vi "Plate Tank 5.vi"() -> ()   [LabVIEW 2019]
uses:
  <vilib>/NI/Current Value Table/Type Defs/Single Tag.ctl
  <vilib>/NI/Current Value Table/Type Defs/Data Types.ctl
  <vilib>/NI/STM/TCP/Read Meta Data (TCP Ref).vi
  <vilib>/NI/STM/TCP/Get Connection Reference (TCP).vi
  <vilib>/NI/AMC/Read Termination Message.vi
  <vilib>/NI/AMC/Create Single Message.vi
  <vilib>/NI/AMC/Update Message Routing Info.vi
  <vilib>/NI/STM/TCP/Read Meta Data (TCP Clst).vi
  <vilib>/NI/AMC/Send Message.vi
  <vilib>/NI/AMC/Globals.vi
  <userlib>/_OpenG.lib/comparison/comparison.llb/I32 Changed__ogtk.vi
  <vilib>/NI/STM/TCP/Write Message (TCP).vi
  <vilib>/NI/AMC/AMC.lvlib
  <vilib>/NI/STM/NI STM.lvlib
  <vilib>/NI/Current Value Table/Current Value Table.lvlib
panel:
  out "Loaded Recipe":string
  in  "Override Motion":bool
  in  "Reverse Current Multiplier":dbl=3.0 min=0.1 max=100.0 step=0.01 format="%.2g"
  in  "Load A Recipe":bool
  in  "Save This Recipe":bool
  out "Right Time":dbl format="%.1f"
  out "Left Time":dbl format="%.1f"
  out "Total Amp*min R":dbl format="%.1f"
  out "Total Amp*min L":dbl format="%.1f"
  in  "Rectifer Settings":i32(listbox)
  in  "MO":string
  in  "BasT1_P Last Hr":bool
  in  "BasT1_Level Last Hr":bool
  out "Boolean 5":bool
  out "SumpBottom":bool
  out "Process 1 Supply":bool
  out "Sump Return":bool
  out "Boolean 2":bool
  out "SG":dbl format="%.3g"
  out "Return to sump 4":bool
  in  "Rectifer Data":enum32{"Standard", "Eng"}(tab)
  out "Current Step":i32
  out "Left Anode Actual Current":dbl(knob) scale=0.0..150.0
  out "Right Anode Actual Current":dbl(knob) scale=0.0..150.0
  out "Left Anode Amp-min":dbl(slide) scale=0.0..800.0
  out "Right Anode Amp-min":dbl(slide) scale=0.0..233.60000610351562
  out "Output Voltage":cluster{dbl, dbl}(graph)
  in  "Tab Control 2":enum32{"Standard", "ENG"}(tab)
  in  "Level Last Hr":bool
  out "Supply Flow":dbl(knob) scale=0.0..65.0
  out "Plating Cell Liquid Level":dbl(slide) scale=0.0..75.0
  out "Cell Temperature":dbl(slide) scale=0.0..60.0
  in  "Cell T Last Hr":bool
  out "Suck Pump":bool
  out "Suck Pump Flow":dbl format="%#_4g"
  out "SuckPipe":bool
  out "SuckPipe 3":bool
  out "Drain Tee Top":bool
  out "Return to sump 2":bool
  out "Return to sump 3":bool
  in  "Supply Tot FlwLast Hr":bool
  in  "Suck FlwLast Hr":bool
  out "Flow Controller":dbl(knob) scale=0.0..100.0
  in  "Tab Control":enum32{"Main Pump", "Suck Pump"}(tab)
  out "Amps":dbl format="%#.2g"
  out "Volts":dbl format="%#.1f"
  out "VFD T":dbl format="%#.2g"
  out "RPM":dbl format="%#.0f"
  out "Fault Code":dbl format="%#.2g"
  out "Freq":dbl format="%#.2g"
  out "SP1 Amps":dbl caption="Amps" format="%#.2g"
  out "SP1 Volts":dbl caption="Volts" format="%#.1g"
  out "SP1 RPM":dbl caption="RPM" format="%#.2g"
  out "SP1 VFD T":dbl caption="VFD T" format="%#.2g"
  out "SP1 Fault Code":dbl caption="Fault Code" format="%#.2g"
  out "SP1 Freq":dbl caption="Freq" format="%#.2g"
  out "Flow 1":dbl format="%#_4g"
  out "Flow 2":dbl format="%#_4g"
  out "Flow 3":dbl format="%#_4g"
  out "Flow 4":dbl format="%#_4g"
  in  "FlowControl Last Hr":bool
  in  "Flow 1 Last Hr":bool
  in  "Flow 2 Last Hr":bool
  in  "Flow 3 Last Hr":bool
  in  "Flow 4 Last Hr":bool
  out "Return to sump":bool
  out "E Stop":bool
  out "Run Enabled?":bool
  in  "Full Drain Plating Cell":bool
  out "Rack Motion":bool
  out "Right Eductor Motion":bool
  out "Left Eductor Motion":bool
  out "Right Output On":bool
  in  "Enable Rack Motion":bool
  in  "Rack RPM":dbl(knob) scale=0.0..15.0
  out "Left Output On":bool
  in  "Start Cycle":bool
  in  "Cancel Cycle":bool
  out "SuckPipe 2":bool
  out "Main Pump":bool
  in  "Enable Eductor Motion":bool
  in  "Eductor RPM":dbl(knob) scale=0.0..15.0
  in  "Supply Pressure (kPa)":dbl(knob)=50.0 min=50.0 max=200.0 step=5.0 scale=50.0..200.0
  in  "Total Inflow (L/min)":dbl(knob)=40.0 min=25.0 max=50.0 step=0.5 scale=25.0..50.0
  in  "Suck Pump fraction of inflow":dbl(knob)=5.0 min=5.0 max=90.0 step=1.0 scale=0.0..90.0
  out "Sump Level":dbl(slide) scale=0.0..1000.0
  out "Supply Pressure":dbl(knob) scale=0.0..200.0
  in  "Enable Suck Pump":bool
  in  "Enable Plating Cell":bool
  in  "Machine":bool
  in  "Basement 4":bool
  in  "Dryer":bool
  in  "Rinse 4":bool
  in  "Rinse 3":bool
  in  "Rinse 2":bool
  in  "Basement 3":bool
  in  "Basement 2":bool
  in  "Basement 1":bool
  in  "Plater 6":bool
  in  "Plater 5":bool
  in  "Plater 4":bool
  in  "Plater 3":bool
  in  "Plater 2":bool
  in  "Plater 1":bool
  in  "Predip":bool
  in  "Rinse 1":bool
  in  "Cleaner":bool
  in  "Etch":bool
  out "status":string
  out "Boolean 4":bool
  # "Module Selection"
  # "Rectifier Settings"
  # "Fluid Flow Control"
  # "Rectifier Control"
  # "Rectifier Output"
  # "Note: RPM settings shared with tank 6"
  # "Motion starts when rectifiers cycle"
  # "kPa"
  # "@"
  # "Output"
  # "cm"
  # "°C"
  # "L/min"
  # "cm"
  # "L/min"
  # "L/min"
  # "L/min"
  # "L/min"
  # "L/min"
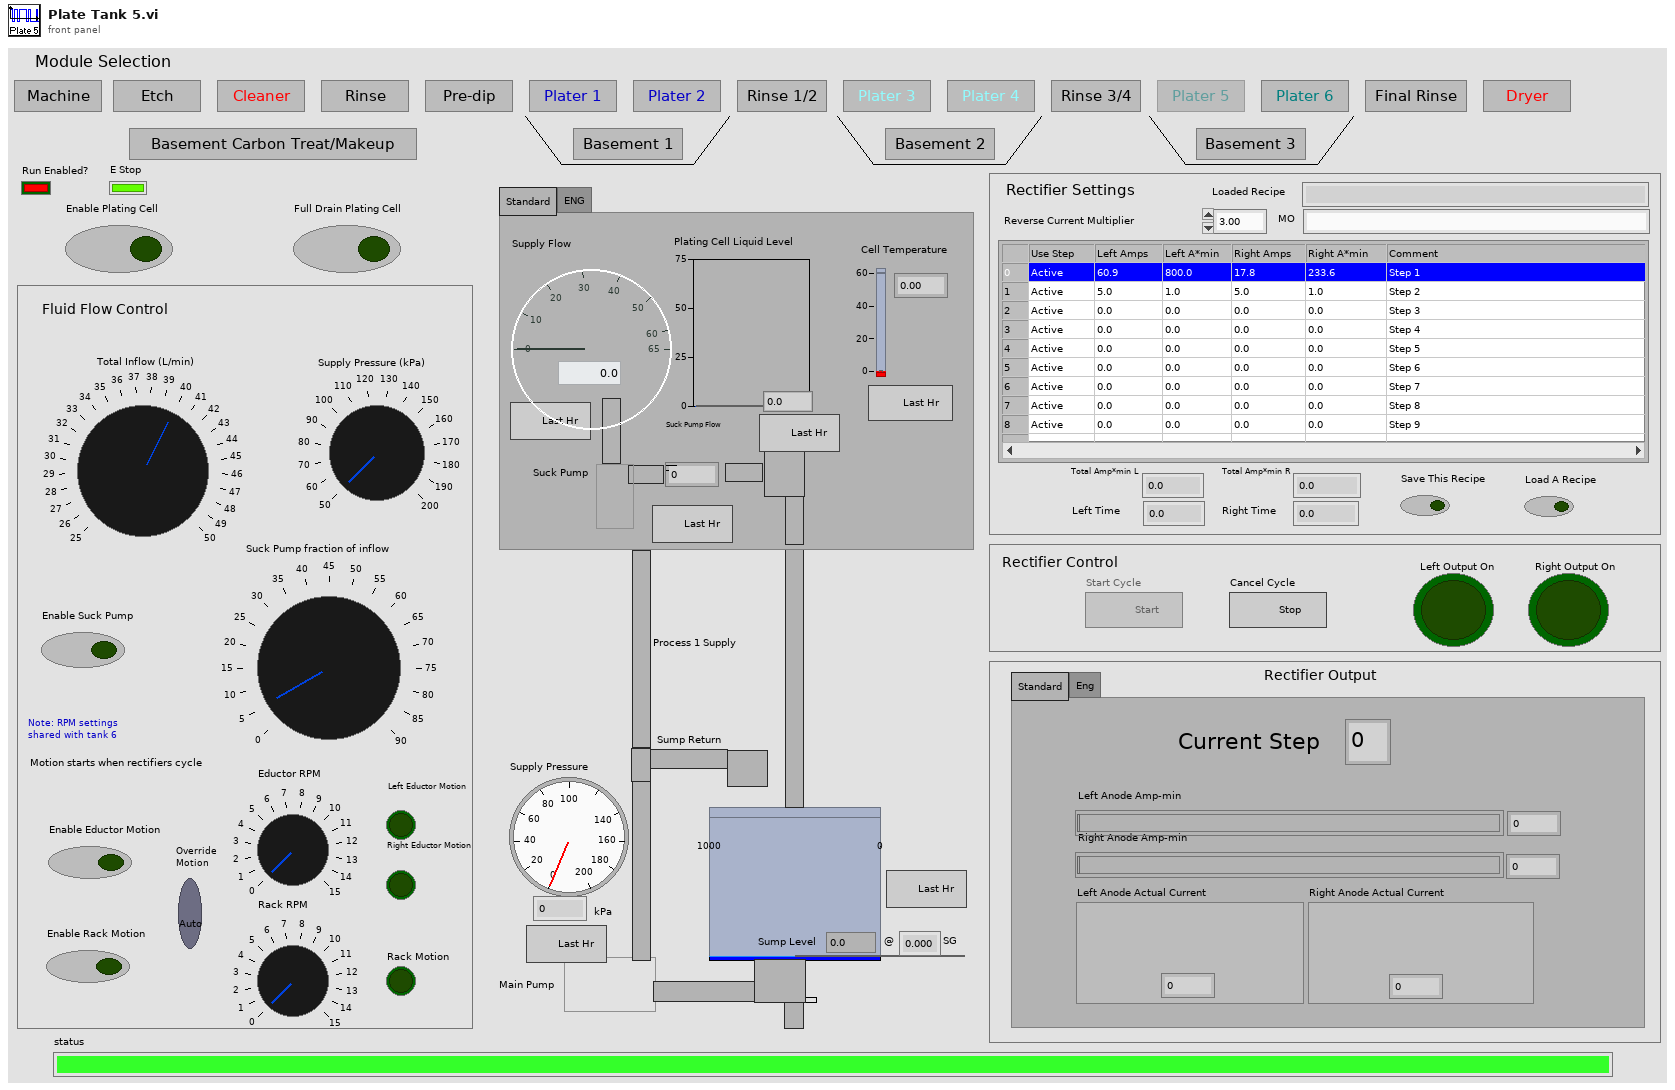
[diagram p1: front panel]
types:
  T1 = typedef "Current Value Table.lvlib/Single Tag.ctl" = cluster{"Data Type":T2, "Name":string, "Value":string, "Description":string}
  T2 = typedef "Current Value Table.lvlib/Data Types.ctl" = enum16{"Double", "Single", "I64", "I32", "I16", "I8", "U64", "U32", "U16", "U8", "String", "Boolean", "Array of U8", "Array of U16", "Array of U32", "Array of U64", "Array of I64", "Array of I32", "Array of I16", "Array of I8", "Array of Double", "Array of Single", "Array of Boolean", "Array of String"}
  T3 = typedef "NI STM.lvlib/TCP Connection Info.ctl" = cluster{"connection ID":refnum<k5>, "meta data":T4[]}
  T4 = typedef "NI STM.lvlib/MetaDataElement.ctl" = string
  T5 = typedef "AMC.lvlib/Message Queue.ctl" = refnum<queue>
  T6 = cluster{"Shift":bool, "Ctrl":bool, "Alt":bool, "Cmd":bool, "Opt":bool}
  T7 = typedef "LVPoint32TypeDef.ctl" = cluster{"Horizontal":i32, "Vertical":i32}
  T8 = typedef "LVRowAndColumnTypeDef.ctl" = cluster{"Row":i32, "Column":i32}
  T9 = enum8{"Enabled", "Disabled", "Disabled and Grayed Out"}
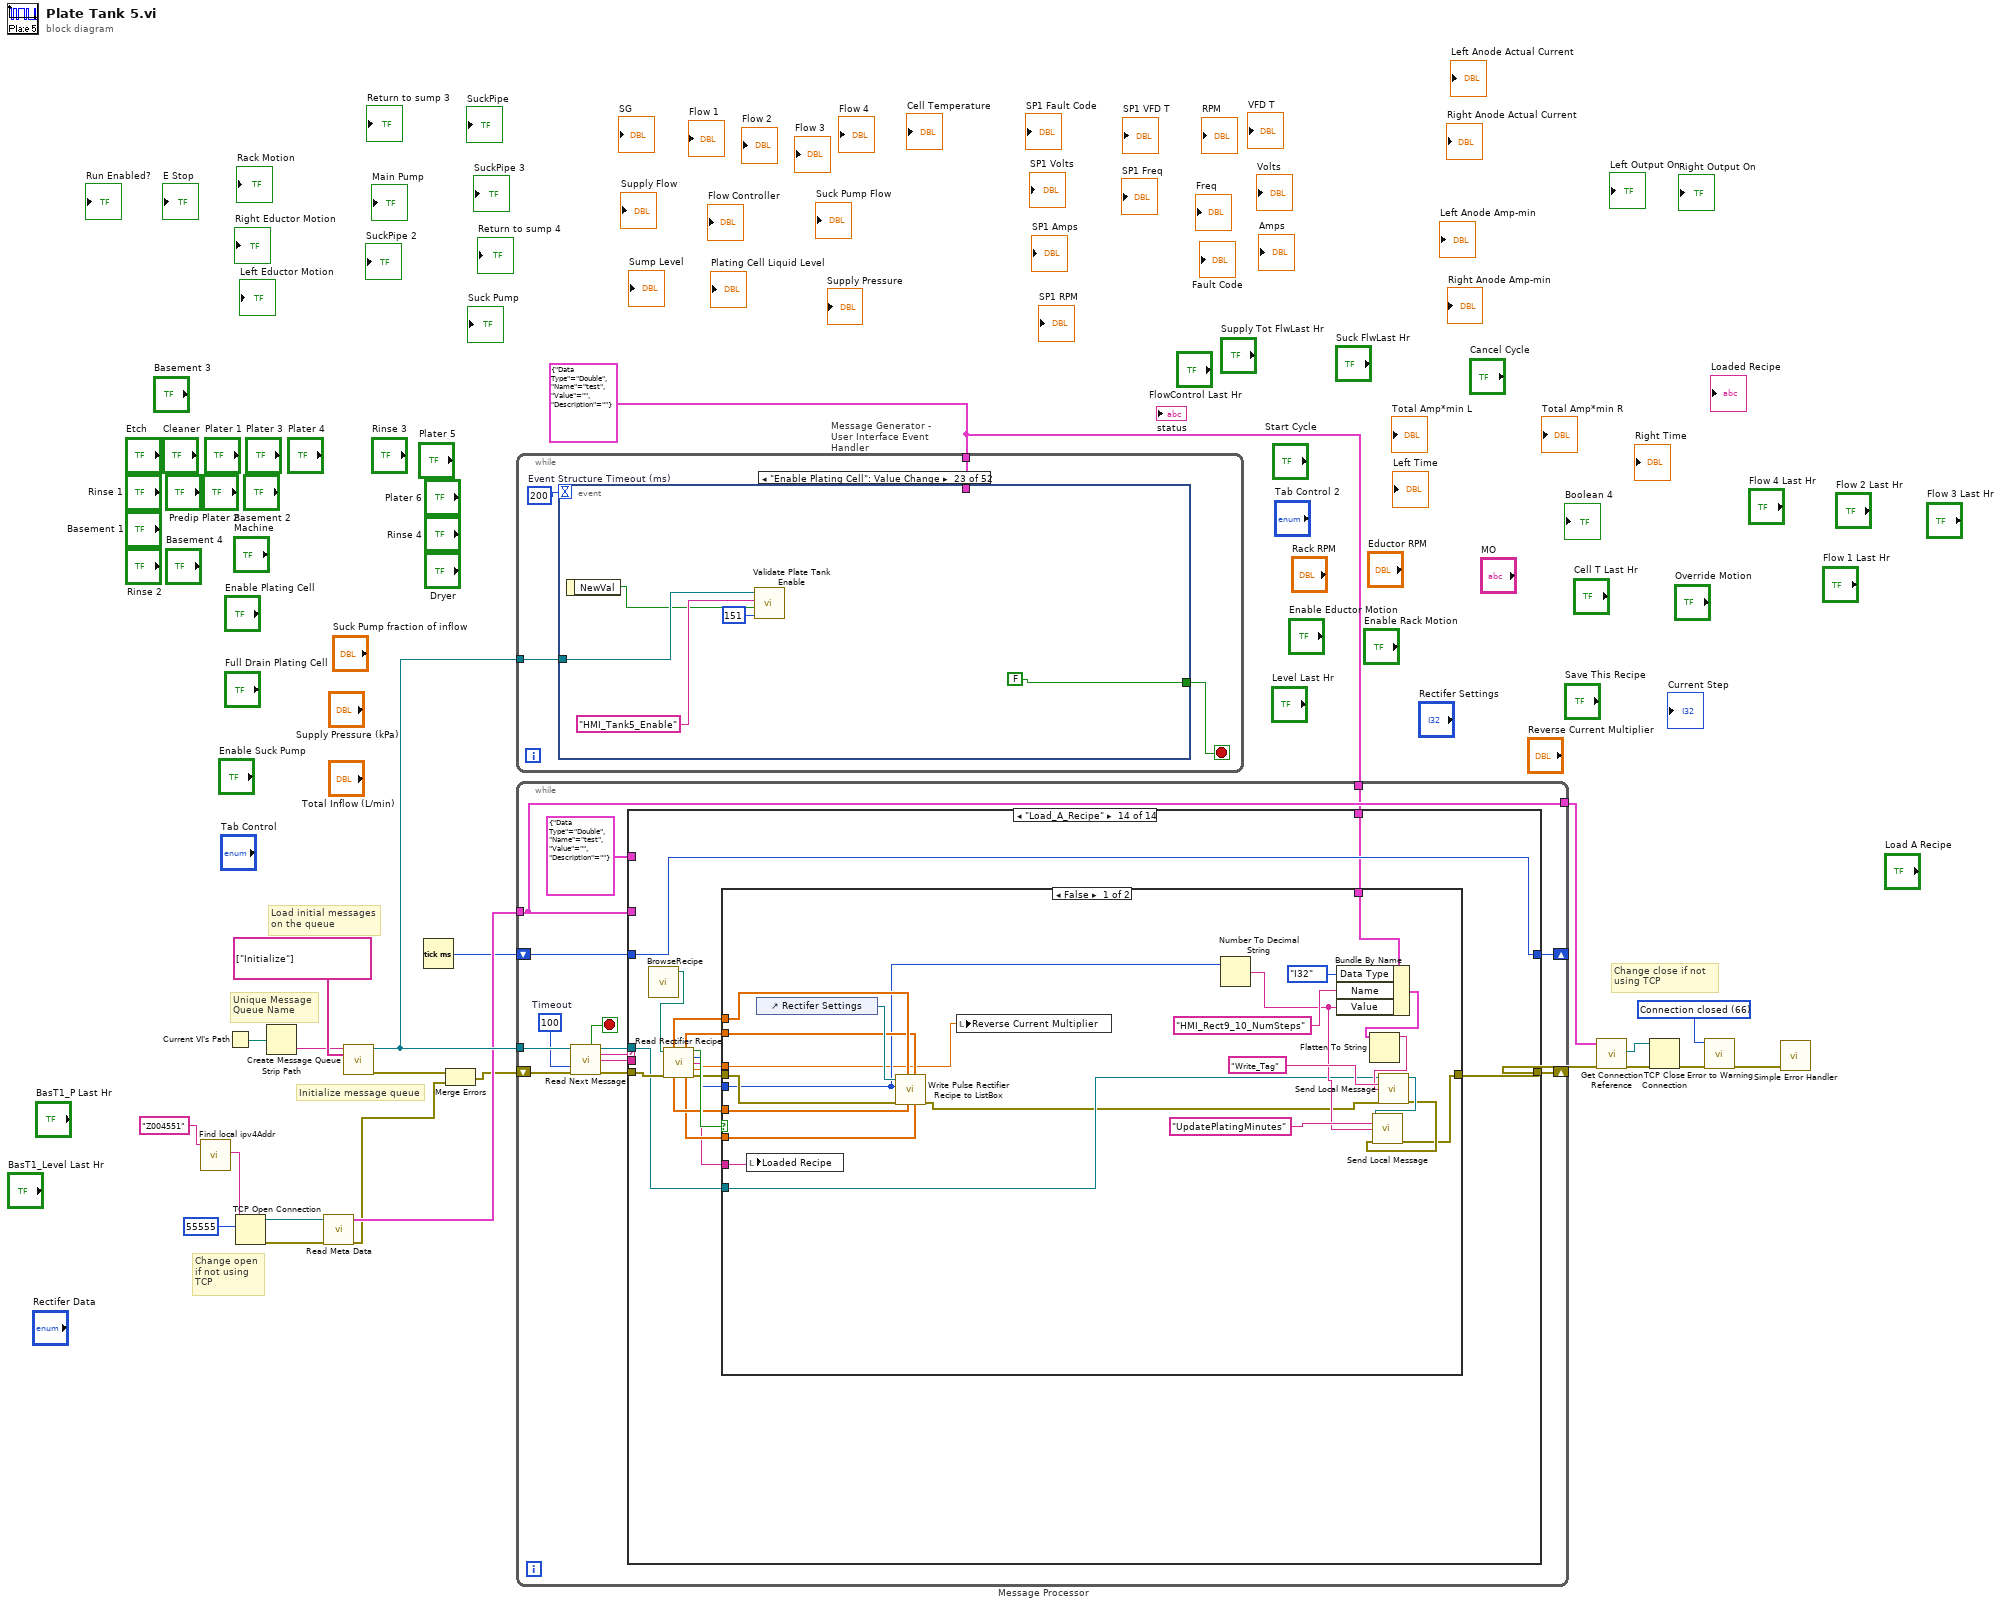
[diagram p0: block diagram]
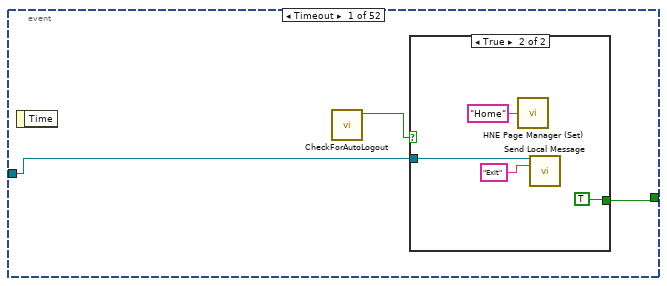
[diagram p2: hidden frame]
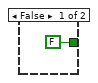
[diagram p3: hidden frame]
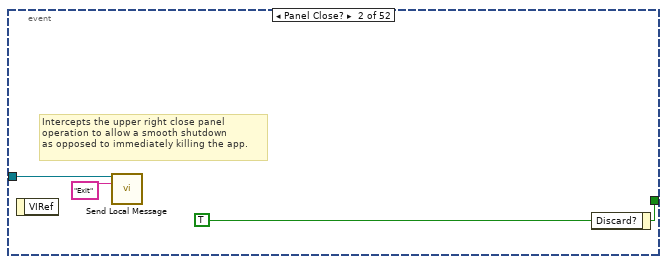
[diagram p4: hidden frame]
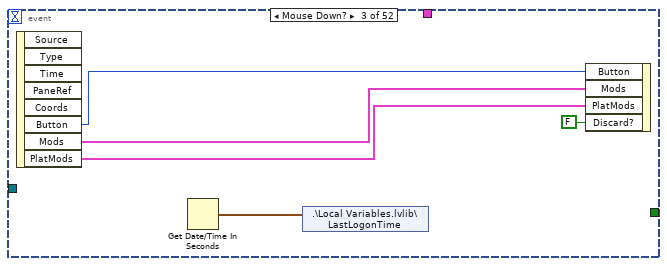
[diagram p5: hidden frame]
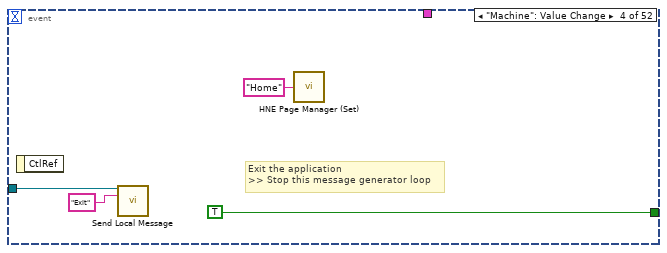
[diagram p6: hidden frame]
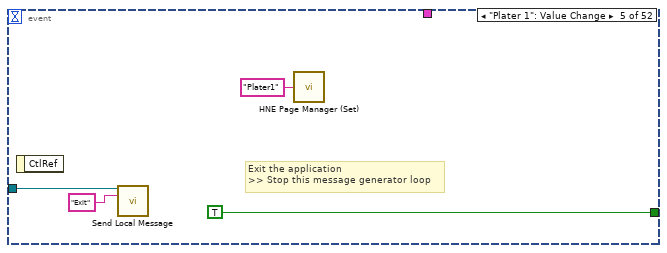
[diagram p7: hidden frame]
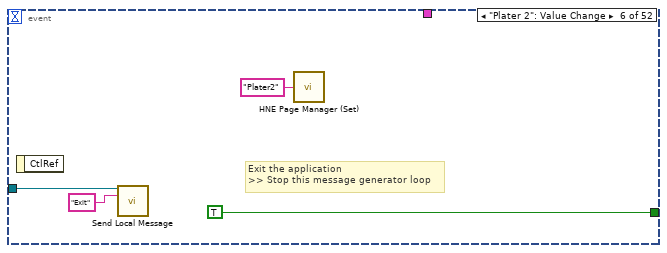
[diagram p8: hidden frame]
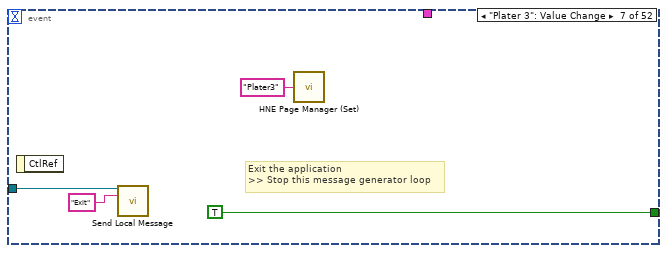
[diagram p9: hidden frame]
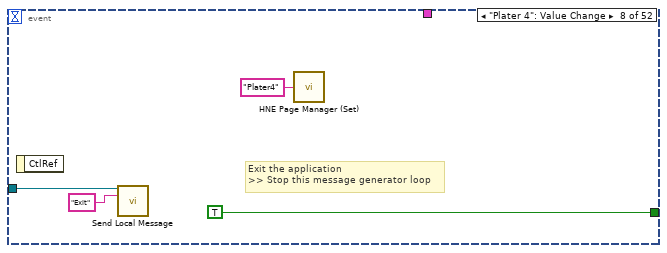
[diagram p10: hidden frame]
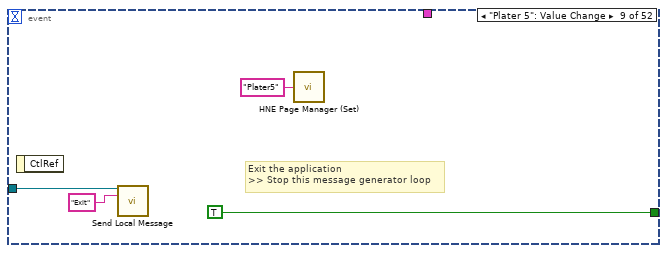
[diagram p11: hidden frame]
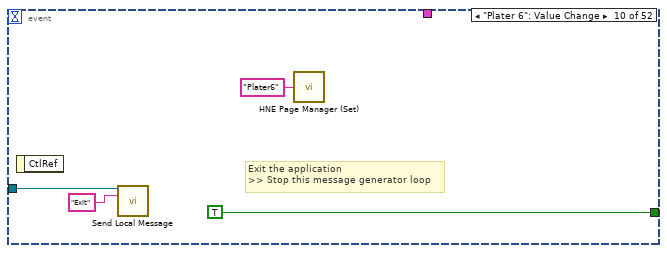
[diagram p12: hidden frame]
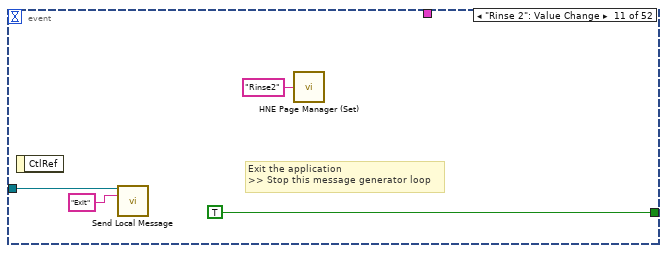
[diagram p13: hidden frame]
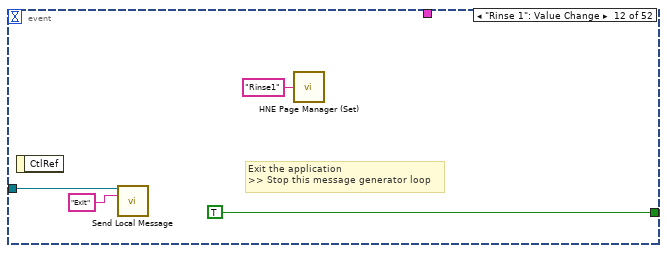
[diagram p14: hidden frame]
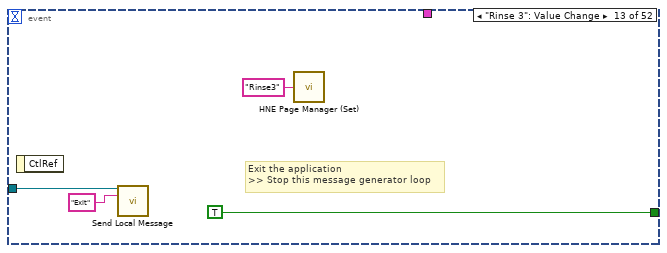
[diagram p15: hidden frame]
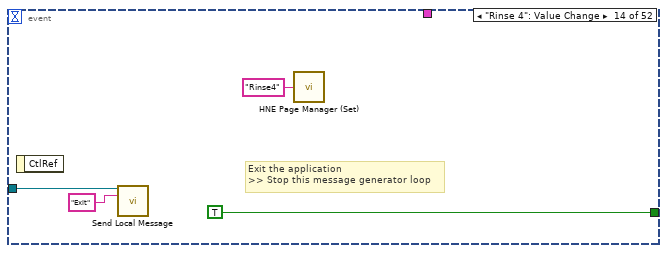
[diagram p16: hidden frame]
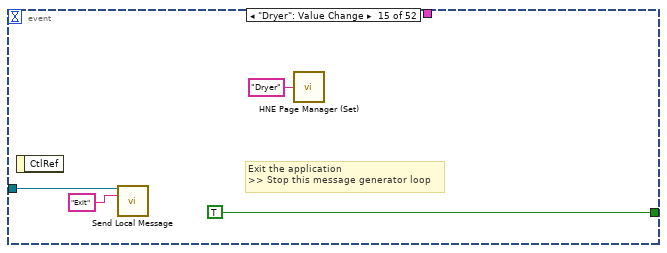
[diagram p17: hidden frame]
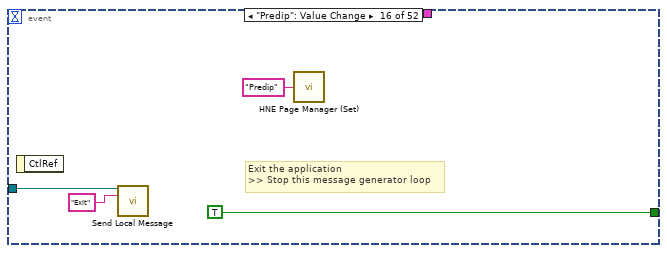
[diagram p18: hidden frame]
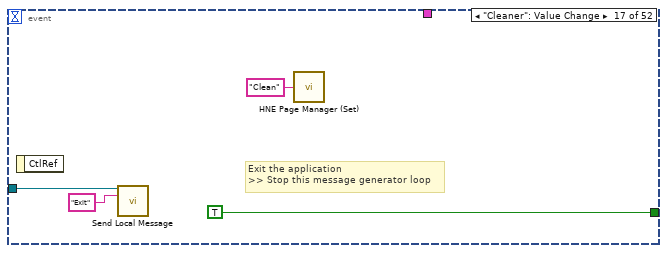
[diagram p19: hidden frame]
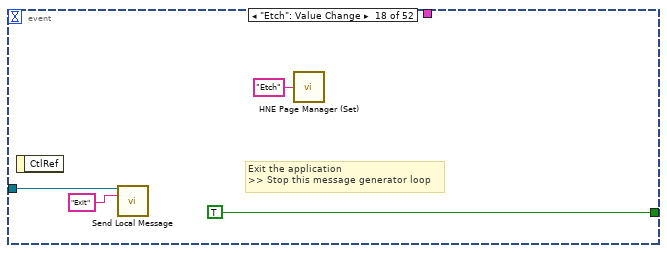
[diagram p20: hidden frame]
diagram:
  w1 = T1 {"Data Type"=enum."Double", "Name"="test", "Value"="", "Description"=""} ("Tag")
  w13 = 66 items=["No Error", "Argument Error", "Memory Full", "Out of Zone", "End of File", "File Already Open", "Generic File IO Error", "File Not Found", "File Permission Error", "Disk Full", "Duplicate Path", "Too Many Files Open", "Not Enabled", "Resource File Not Found", "Cannot Add Resource", "Resource Not Found", "Image Not Found", "Image Memory Error", "Pen Does Not Exist", "Config Bad Type", "Config Token Not Found", "Config Parse Error", "Config Memory Error", "Bad External Code Format", "Bad External Code Offset", "External Code Not Present", "Null Window", "Destroy Window Mixup", "Null Menu", "Print Aborted", "Bad Print Record", "Print Driver Error", "Windows Error During Print", "Memory Error During Print", "Print Dialog Error", "Generic Print Error", "Invalid Device Refnum", "Device Not Found", "Device Parameter Error", "Device Unit Error", "Can't Open Device", "Device Call Aborted", "Generic Error", "Cancelled By User", "Object ID Too Low", "Object ID Too High", "Object Not In Heap", "Unknown Heap", "Bad DefProc ID", "DefProc Not In Table", "Message Out Of Range", "Null Method", "Unknown Message", "Manager Call Not Supported", "Bad address", "Connection In progress", "Connection timed out", "Connection is already in progress", "Network attribute not supported", "Network error", "Address in use", "System out of memory", "Connection aborted", "Connection refused", "Connection is not connected", "Connection is already connected", "Connection closed", "Initialize error (interapplication manager)", "Bad occurrence", "Wait on unbound occurrence handler", "Occurrence queue overflow", "Bad path", "Semaphore not signaled", "Unrecognized type (interapplication manager)"] ("1st Error to Convert")
  # "Change close if not using TCP"
  # "Change open if not using TCP"
  # "Initialize message queue"
  # "Unique Message\nQueue Name"
  # "Load initial messages\non the queue"
  n1 = call "Find local ipv4Addr.vi"("MachineToFind"="Z004551" ("Target IP Address")) -> ("name"=w5:string)  [unwired: 9 in, 1 out]
  n2 = Current VI's Path() -> (path=w19:path)
  n3 = TCP Open Connection(address=w5, remote port or service name=u16 55555 ("remote port")) -> (connection ID=w17:refnum<k5>, error out=w16:errorcluster)  [unwired: 1 in, 2 out]
  n4 = Strip Path(path=w19) -> (name=w21:string)  [unwired: 1 out]
  n5 = call-poly <vilib>:"Read Meta Data.vi"("error in"=w16, "connection ID"=w17) -> ("error out"=w3:errorcluster, "connection info out"=w15:T3)  [unwired: 7 in, 1 out]
  n6 = call <vilib>:"Create Message Queue.vi"("message queue name"=w21, "initial message names"=string[] ["Initialize"]) -> ("message queue out"=w20:T5, "error out"=w4:errorcluster)  [unwired: 12 in]
  n7 = Tick Count (ms)() -> (millisecond timer value=w7:u32)
  n8 = Merge Errors(w4, w3) -> (w2:errorcluster)
  n9 = while "Message Generator - User Interface Event Handler" {
    tunnel: w20 -> [w24]
    tunnel: w1 -> [w23]
    stop <- w25 stop-if-true
    w26 = 200  # Event Structure Timeout (ms)
    n10 = event shown="[22] \"Enable Plating Cell\": Value Change" {
      selector: _ -> [_ _ _ _ _ _ _ _ _ _ _ _ _ _ _ _ _ _ _ _ _ _ _ _ _ _ _ _ _ _ _ _ _ _ _ _ _ _ _ _ _ _ _ _ _ _ _ _ _ _ _ _]
      dyn-events: _ -> [_ _ _ _ _ _ _ _ _ _ _ _ _ _ _ _ _ _ _ _ _ _ _ _ _ _ _ _ _ _ _ _ _ _ _ _ _ _ _ _ _ _ _ _ _ _ _ _ _ _ _ _]
      timeout: w26 -> [_ _ _ _ _ _ _ _ _ _ _ _ _ _ _ _ _ _ _ _ _ _ _ _ _ _ _ _ _ _ _ _ _ _ _ _ _ _ _ _ _ _ _ _ _ _ _ _ _ _ _ _]
      tunnel: [w29 w37 _ TRUE ("Discard?") TRUE ("Discard?") TRUE ("Discard?") TRUE ("Discard?") TRUE ("Discard?") TRUE ("Discard?") TRUE ("Discard?") TRUE ("Discard?") TRUE ("Discard?") TRUE ("Discard?") TRUE ("Discard?") TRUE ("Discard?") TRUE ("Discard?") TRUE ("Discard?") TRUE ("Discard?") TRUE ("Discard?") TRUE ("Discard?") TRUE ("Discard?") TRUE ("Discard?") FALSE ("Discard?") FALSE ("Discard?") FALSE ("Discard?") FALSE ("Discard?") FALSE ("Discard?") FALSE ("Discard?") FALSE ("Discard?") FALSE ("Discard?") FALSE ("Discard?") FALSE ("Discard?") FALSE ("Discard?") FALSE ("Discard?") FALSE ("Discard?") FALSE ("Discard?") FALSE ("Discard?") _ _ _ _ _ _ _ _ _ _ _ _ _ _ _] -> w25
      tunnel: w24 -> [w28 w35 _ w44 w48 w52 w56 w60 w64 w68 w72 w76 w80 w84 w88 w92 w96 w100 w104 w108 w112 w116 w122 w125 w130 w143 w154 w165 w176 w187 w191 w205 w225 w235 w245 w255 w267 w269 w271 w276 w281 w286 w291 w296 w301 w306 w311 w316 w321 w328 w346 _]
      tunnel: w23 -> [_ _ _ _ _ _ _ _ _ _ _ _ _ _ _ _ _ _ _ _ _ _ _ _ _ w140 w151 w162 w173 w184 w190 w204 w224 w234 w244 w254 w266 _ _ _ _ _ _ _ _ _ _ _ _ w327 _ _]
      event Timeout {
        n11 = event-data() -> ()  [unwired: 2 out]
        n12 = call "CheckForAutoLogout.vi"() -> ("Boolean"=w27:bool)  [unwired: 11 in]
        n13 = case shown="True" w27 {
          tunnel: [FALSE ("Discard?") TRUE ("Discard?")] -> w29
          tunnel: w28 -> [_ w31]
          frame False {
          }
          frame True {
            n14 = call <userlib>:"HNE Page Manager (Set).vi"("Next Page"="Home") -> ()  [unwired: 4 in, 1 out]
            n15 = call <vilib>:"Send Local Message.vi"("message queue in"=w31, "message name"="Exit") -> ()  [unwired: 11 in, 3 out]
          }
        }
      }
      event Panel Close? {
        w37 = TRUE ("Discard?")
        # "Intercepts the upper right close panel\noperation to allow a smooth shutdown\nas opposed to immediately killing the app."
        n16 = event-data() -> ()  [unwired: 2 out]
        n17 = call <vilib>:"Send Local Message.vi"("message queue in"=w35, "message name"="Exit") -> ()  [unwired: 11 in, 3 out]
        n18 = event-data("Discard?"=w37) -> ()  [unwired: 1 in, 1 out]
      }
      event Mouse Down? {
        n19 = event-data() -> ("Button"=w41:u16, "Mods"=w40:cluster{"Double Click":bool, "Menu Key":bool}, "PlatMods"=w39:T6)  [unwired: 6 out]
        n20 = Get Date/Time In Seconds() -> (seconds since 1Jan1904=w38:timestamp)
        n21 = shared-variable ".\\Local Variables.lvlib\\LastLogonTime"(w38) -> ()  [unwired: 1 in, 1 out]
        n22 = event-data("Button"=w41, "Mods"=w40, "PlatMods"=w39, "Discard?"=FALSE) -> ()  [unwired: 1 in, 1 out]
      }
      event "Machine": Value Change {
        # "Exit the application\n>> Stop this message generator loop"
        n23 = event-data() -> ()  [unwired: 2 out]
        n24 = call <vilib>:"Send Local Message.vi"("message queue in"=w44, "message name"="Exit") -> ()  [unwired: 11 in, 3 out]
        n25 = call <userlib>:"HNE Page Manager (Set).vi"("Next Page"="Home") -> ()  [unwired: 4 in, 1 out]
      }
      event "Plater 1": Value Change {
        # "Exit the application\n>> Stop this message generator loop"
        n26 = event-data() -> ()  [unwired: 2 out]
        n27 = call <vilib>:"Send Local Message.vi"("message queue in"=w48, "message name"="Exit") -> ()  [unwired: 11 in, 3 out]
        n28 = call <userlib>:"HNE Page Manager (Set).vi"("Next Page"="Plater1") -> ()  [unwired: 4 in, 1 out]
      }
      event "Plater 2": Value Change {
        # "Exit the application\n>> Stop this message generator loop"
        n29 = event-data() -> ()  [unwired: 2 out]
        n30 = call <vilib>:"Send Local Message.vi"("message queue in"=w52, "message name"="Exit") -> ()  [unwired: 11 in, 3 out]
        n31 = call <userlib>:"HNE Page Manager (Set).vi"("Next Page"="Plater2") -> ()  [unwired: 4 in, 1 out]
      }
      event "Plater 3": Value Change {
        # "Exit the application\n>> Stop this message generator loop"
        n32 = event-data() -> ()  [unwired: 2 out]
        n33 = call <vilib>:"Send Local Message.vi"("message queue in"=w56, "message name"="Exit") -> ()  [unwired: 11 in, 3 out]
        n34 = call <userlib>:"HNE Page Manager (Set).vi"("Next Page"="Plater3") -> ()  [unwired: 4 in, 1 out]
      }
      event "Plater 4": Value Change {
        # "Exit the application\n>> Stop this message generator loop"
        n35 = event-data() -> ()  [unwired: 2 out]
        n36 = call <vilib>:"Send Local Message.vi"("message queue in"=w60, "message name"="Exit") -> ()  [unwired: 11 in, 3 out]
        n37 = call <userlib>:"HNE Page Manager (Set).vi"("Next Page"="Plater4") -> ()  [unwired: 4 in, 1 out]
      }
      event "Plater 5": Value Change {
        # "Exit the application\n>> Stop this message generator loop"
        n38 = event-data() -> ()  [unwired: 2 out]
        n39 = call <vilib>:"Send Local Message.vi"("message queue in"=w64, "message name"="Exit") -> ()  [unwired: 11 in, 3 out]
        n40 = call <userlib>:"HNE Page Manager (Set).vi"("Next Page"="Plater5") -> ()  [unwired: 4 in, 1 out]
      }
      event "Plater 6": Value Change {
        # "Exit the application\n>> Stop this message generator loop"
        n41 = event-data() -> ()  [unwired: 2 out]
        n42 = call <vilib>:"Send Local Message.vi"("message queue in"=w68, "message name"="Exit") -> ()  [unwired: 11 in, 3 out]
        n43 = call <userlib>:"HNE Page Manager (Set).vi"("Next Page"="Plater6") -> ()  [unwired: 4 in, 1 out]
      }
      event "Rinse 2": Value Change {
        # "Exit the application\n>> Stop this message generator loop"
        n44 = event-data() -> ()  [unwired: 2 out]
        n45 = call <vilib>:"Send Local Message.vi"("message queue in"=w72, "message name"="Exit") -> ()  [unwired: 11 in, 3 out]
        n46 = call <userlib>:"HNE Page Manager (Set).vi"("Next Page"="Rinse2") -> ()  [unwired: 4 in, 1 out]
      }
      event "Rinse 1": Value Change {
        # "Exit the application\n>> Stop this message generator loop"
        n47 = event-data() -> ()  [unwired: 2 out]
        n48 = call <vilib>:"Send Local Message.vi"("message queue in"=w76, "message name"="Exit") -> ()  [unwired: 11 in, 3 out]
        n49 = call <userlib>:"HNE Page Manager (Set).vi"("Next Page"="Rinse1") -> ()  [unwired: 4 in, 1 out]
      }
      event "Rinse 3": Value Change {
        # "Exit the application\n>> Stop this message generator loop"
        n50 = event-data() -> ()  [unwired: 2 out]
        n51 = call <vilib>:"Send Local Message.vi"("message queue in"=w80, "message name"="Exit") -> ()  [unwired: 11 in, 3 out]
        n52 = call <userlib>:"HNE Page Manager (Set).vi"("Next Page"="Rinse3") -> ()  [unwired: 4 in, 1 out]
      }
      event "Rinse 4": Value Change {
        # "Exit the application\n>> Stop this message generator loop"
        n53 = event-data() -> ()  [unwired: 2 out]
        n54 = call <vilib>:"Send Local Message.vi"("message queue in"=w84, "message name"="Exit") -> ()  [unwired: 11 in, 3 out]
        n55 = call <userlib>:"HNE Page Manager (Set).vi"("Next Page"="Rinse4") -> ()  [unwired: 4 in, 1 out]
      }
      event "Dryer": Value Change {
        # "Exit the application\n>> Stop this message generator loop"
        n56 = event-data() -> ()  [unwired: 2 out]
        n57 = call <vilib>:"Send Local Message.vi"("message queue in"=w88, "message name"="Exit") -> ()  [unwired: 11 in, 3 out]
        n58 = call <userlib>:"HNE Page Manager (Set).vi"("Next Page"="Dryer") -> ()  [unwired: 4 in, 1 out]
      }
      event "Predip": Value Change {
        # "Exit the application\n>> Stop this message generator loop"
        n59 = event-data() -> ()  [unwired: 2 out]
        n60 = call <vilib>:"Send Local Message.vi"("message queue in"=w92, "message name"="Exit") -> ()  [unwired: 11 in, 3 out]
        n61 = call <userlib>:"HNE Page Manager (Set).vi"("Next Page"="Predip") -> ()  [unwired: 4 in, 1 out]
      }
      event "Cleaner": Value Change {
        # "Exit the application\n>> Stop this message generator loop"
        n62 = event-data() -> ()  [unwired: 2 out]
        n63 = call <vilib>:"Send Local Message.vi"("message queue in"=w96, "message name"="Exit") -> ()  [unwired: 11 in, 3 out]
        n64 = call <userlib>:"HNE Page Manager (Set).vi"("Next Page"="Clean") -> ()  [unwired: 4 in, 1 out]
      }
      event "Etch": Value Change {
        # "Exit the application\n>> Stop this message generator loop"
        n65 = event-data() -> ()  [unwired: 2 out]
        n66 = call <vilib>:"Send Local Message.vi"("message queue in"=w100, "message name"="Exit") -> ()  [unwired: 11 in, 3 out]
        n67 = call <userlib>:"HNE Page Manager (Set).vi"("Next Page"="Etch") -> ()  [unwired: 4 in, 1 out]
      }
      event "Basement 1": Value Change {
        # "Exit the application\n>> Stop this message generator loop"
        n68 = event-data() -> ()  [unwired: 2 out]
        n69 = call <vilib>:"Send Local Message.vi"("message queue in"=w104, "message name"="Exit") -> ()  [unwired: 11 in, 3 out]
        n70 = call <userlib>:"HNE Page Manager (Set).vi"("Next Page"="Basement1") -> ()  [unwired: 4 in, 1 out]
      }
      event "Basement 2": Value Change {
        # "Exit the application\n>> Stop this message generator loop"
        n71 = event-data() -> ()  [unwired: 2 out]
        n72 = call <vilib>:"Send Local Message.vi"("message queue in"=w108, "message name"="Exit") -> ()  [unwired: 11 in, 3 out]
        n73 = call <userlib>:"HNE Page Manager (Set).vi"("Next Page"="Basement2") -> ()  [unwired: 4 in, 1 out]
      }
      event "Basement 3": Value Change {
        # "Exit the application\n>> Stop this message generator loop"
        n74 = event-data() -> ()  [unwired: 2 out]
        n75 = call <vilib>:"Send Local Message.vi"("message queue in"=w112, "message name"="Exit") -> ()  [unwired: 11 in, 3 out]
        n76 = call <userlib>:"HNE Page Manager (Set).vi"("Next Page"="Basement3") -> ()  [unwired: 4 in, 1 out]
      }
      event "Basement 4": Value Change {
        # "Exit the application\n>> Stop this message generator loop"
        n77 = event-data() -> ()  [unwired: 2 out]
        n78 = call <vilib>:"Send Local Message.vi"("message queue in"=w116, "message name"="Exit") -> ()  [unwired: 11 in, 3 out]
        n79 = call <userlib>:"HNE Page Manager (Set).vi"("Next Page"="Basement4") -> ()  [unwired: 4 in, 1 out]
      }
      event "Enable Plating Cell": Value Change {
        n80 = event-data() -> ("NewVal"=w120:bool)  [unwired: 1 out]
        n81 = call "Validate Plate Tank Enable.vi"("Valve No."=151, "Test Value"=w120, "Tag"="HMI_Tank5_Enable", "Queue in"=w122) -> ()  [unwired: 8 in]
      }
      event "Save This Recipe": Value Change {
        n82 = event-data() -> ("NewVal"=w124:bool)  [unwired: 1 out]
        n83 = case shown="True" w124 {
          tunnel: w125 -> [_ w127]
          frame False {
          }
          frame True {
            n84 = call <vilib>:"Send Local Message.vi"("message queue in"=w127, "message name"="Save_Recipe") -> ()  [unwired: 11 in, 3 out]
          }
        }
      }
      event "Load A Recipe": Value Change {
        n85 = event-data() -> ("NewVal"=w129:bool)  [unwired: 1 out]
        n86 = case shown="True" w129 {
          tunnel: w130 -> [_ w132]
          frame False {
          }
          frame True {
            n87 = call <vilib>:"Send Local Message.vi"("message queue in"=w132, "message name"="Load_A_Recipe") -> ()  [unwired: 11 in, 3 out]
          }
        }
      }
      event "Full Drain Plating Cell": Value Change {
        n88 = event-data() -> ("NewVal"=w142:bool)  [unwired: 1 out]
        n89 = Boolean To (0,1)(Boolean=w142) -> (0, 1=w141:i16)
        n90 = Number To Decimal String(number=w141) -> (decimal integer string=w137:string)  [unwired: 1 in]
        n91 = Bundle By Name(cluster=w140, "Data Type"=Data_Types."Boolean", "Name"="HMI_Tank5_Drain", "Value"=w137) -> (w136:T1)
        n92 = Flatten To String(anything=w136) -> (data string=w135:string)  [unwired: 3 in, 2 out]
        n93 = call <vilib>:"Send Local Message.vi"("message queue in"=w143, "message name"="Write_Tag", "message value"=w135) -> ()  [unwired: 10 in, 3 out]
      }
      event "Enable Eductor Motion": Value Change {
        n94 = event-data() -> ("NewVal"=w153:bool)  [unwired: 1 out]
        n95 = Boolean To (0,1)(Boolean=w153) -> (0, 1=w152:i16)
        n96 = Number To Decimal String(number=w152) -> (decimal integer string=w148:string)  [unwired: 1 in]
        n97 = Bundle By Name(cluster=w151, "Data Type"=Data_Types."Boolean", "Name"="HMI_Tank5_Eductor_Motors_Run", "Value"=w148) -> (w147:T1)
        n98 = Flatten To String(anything=w147) -> (data string=w146:string)  [unwired: 3 in, 2 out]
        n99 = call <vilib>:"Send Local Message.vi"("message queue in"=w154, "message name"="Write_Tag", "message value"=w146) -> ()  [unwired: 10 in, 3 out]
      }
      event "Enable Rack Motion": Value Change {
        n100 = event-data() -> ("NewVal"=w164:bool)  [unwired: 1 out]
        n101 = Boolean To (0,1)(Boolean=w164) -> (0, 1=w163:i16)
        n102 = Number To Decimal String(number=w163) -> (decimal integer string=w159:string)  [unwired: 1 in]
        n103 = Bundle By Name(cluster=w162, "Data Type"=Data_Types."Boolean", "Name"="HMI_Tank5_Rack_Motor_Run", "Value"=w159) -> (w158:T1)
        n104 = Flatten To String(anything=w158) -> (data string=w157:string)  [unwired: 3 in, 2 out]
        n105 = call <vilib>:"Send Local Message.vi"("message queue in"=w165, "message name"="Write_Tag", "message value"=w157) -> ()  [unwired: 10 in, 3 out]
      }
      event "Enable Suck Pump": Value Change {
        n106 = event-data() -> ("NewVal"=w175:bool)  [unwired: 1 out]
        n107 = Boolean To (0,1)(Boolean=w175) -> (0, 1=w174:i16)
        n108 = Number To Decimal String(number=w174) -> (decimal integer string=w170:string)  [unwired: 1 in]
        n109 = Bundle By Name(cluster=w173, "Data Type"=Data_Types."Boolean", "Name"="HMI_Tnk5_Enable_SuckPump", "Value"=w170) -> (w169:T1)
        n110 = Flatten To String(anything=w169) -> (data string=w168:string)  [unwired: 3 in, 2 out]
        n111 = call <vilib>:"Send Local Message.vi"("message queue in"=w176, "message name"="Write_Tag", "message value"=w168) -> ()  [unwired: 10 in, 3 out]
      }
      event "Override Motion": Value Change {
        n112 = event-data() -> ("NewVal"=w186:bool)  [unwired: 1 out]
        n113 = Boolean To (0,1)(Boolean=w186) -> (0, 1=w185:i16)
        n114 = Number To Decimal String(number=w185) -> (decimal integer string=w181:string)  [unwired: 1 in]
        n115 = Bundle By Name(cluster=w184, "Data Type"=Data_Types."Boolean", "Name"="HMI_Tank5_Motion_OverRide", "Value"=w181) -> (w180:T1)
        n116 = Flatten To String(anything=w180) -> (data string=w179:string)  [unwired: 3 in, 2 out]
        n117 = call <vilib>:"Send Local Message.vi"("message queue in"=w187, "message name"="Write_Tag", "message value"=w179) -> ()  [unwired: 10 in, 3 out]
      }
      event "Start Cycle": Value Change {
        n118 = event-data() -> ("NewVal"=w189:bool)  [unwired: 1 out]
        n119 = case shown="True" w189 {
          tunnel: w191 -> [_ w202]
          tunnel: w189 -> [_ w201]
          tunnel: w190 -> [_ w199]
          frame False {
          }
          frame True {
            n120 = Boolean To (0,1)(Boolean=w201) -> (0, 1=w200:i16)
            n121 = Number To Decimal String(number=w200) -> (decimal integer string=w196:string)  [unwired: 1 in]
            n122 = Bundle By Name(cluster=w199, "Data Type"=Data_Types."Boolean", "Name"="HMI_Rect9_10_Cycle", "Value"=w196) -> (w195:T1)
            n123 = Flatten To String(anything=w195) -> (data string=w194:string)  [unwired: 3 in, 2 out]
            n124 = call <vilib>:"Send Local Message.vi"("message queue in"=w202, "message name"="Write_Tag", "message value"=w194) -> ()  [unwired: 10 in, 3 out]
          }
        }
      }
      event "Cancel Cycle": Value Change {
        n125 = event-data() -> ("NewVal"=w203:bool)  [unwired: 1 out]
        n126 = case shown="True" w203 {
          tunnel: w205 -> [_ w216]
          tunnel: w203 -> [_ w215]
          tunnel: w204 -> [_ w213]
          frame False {
          }
          frame True {
            n127 = Boolean To (0,1)(Boolean=w215) -> (0, 1=w214:i16)
            n128 = Number To Decimal String(number=w214) -> (decimal integer string=w210:string)  [unwired: 1 in]
            n129 = Bundle By Name(cluster=w213, "Data Type"=Data_Types."Boolean", "Name"="HMI_Rect9_10_CycleStop", "Value"=w210) -> (w209:T1)
            n130 = Flatten To String(anything=w209) -> (data string=w208:string)  [unwired: 3 in, 2 out]
            n131 = call <vilib>:"Send Local Message.vi"("message queue in"=w216, "message name"="Write_Tag", "message value"=w208) -> ()  [unwired: 10 in, 3 out]
          }
        }
      }
      event "Eductor RPM": Value Change {
        n132 = event-data() -> ("NewVal"=w218:dbl)  [unwired: 1 out]
        n133 = Number To Fractional String(number=w218) -> (F-format string=w217:string)  [unwired: 3 in]
        n134 = Bundle By Name(cluster=w224, "Data Type"=Data_Types."Double", "Name"="HMI_Tnk5_Eductor_RPM", "Value"=w217) -> (w221:T1)
        n135 = Flatten To String(anything=w221) -> (data string=w220:string)  [unwired: 3 in, 2 out]
        n136 = call <vilib>:"Send Local Message.vi"("message queue in"=w225, "message name"="Write_Tag", "message value"=w220) -> ()  [unwired: 10 in, 3 out]
      }
      event "Rack RPM": Value Change {
        n137 = event-data() -> ("NewVal"=w228:dbl)  [unwired: 1 out]
        n138 = Number To Fractional String(number=w228) -> (F-format string=w227:string)  [unwired: 3 in]
        n139 = Bundle By Name(cluster=w234, "Data Type"=Data_Types."Double", "Name"="HMI_Tnk5_Rack_RPM", "Value"=w227) -> (w231:T1)
        n140 = Flatten To String(anything=w231) -> (data string=w230:string)  [unwired: 3 in, 2 out]
        n141 = call <vilib>:"Send Local Message.vi"("message queue in"=w235, "message name"="Write_Tag", "message value"=w230) -> ()  [unwired: 10 in, 3 out]
      }
      event "Total Inflow (L/min)": Value Change {
        n142 = event-data() -> ("NewVal"=w238:dbl)  [unwired: 1 out]
        n143 = Number To Fractional String(number=w238) -> (F-format string=w237:string)  [unwired: 3 in]
        n144 = Bundle By Name(cluster=w244, "Data Type"=Data_Types."Double", "Name"="HMI_TNK5_Flow_Setpoint", "Value"=w237) -> (w241:T1)
        n145 = Flatten To String(anything=w241) -> (data string=w240:string)  [unwired: 3 in, 2 out]
        n146 = call <vilib>:"Send Local Message.vi"("message queue in"=w245, "message name"="Write_Tag", "message value"=w240) -> ()  [unwired: 10 in, 3 out]
      }
      event "Supply Pressure (kPa)": Value Change {
        n147 = event-data() -> ("NewVal"=w248:dbl)  [unwired: 1 out]
        n148 = Number To Fractional String(number=w248) -> (F-format string=w247:string)  [unwired: 3 in]
        n149 = Bundle By Name(cluster=w254, "Data Type"=Data_Types."Double", "Name"="HMI_BAS_TNK3_P_Setpoint", "Value"=w247) -> (w251:T1)
        n150 = Flatten To String(anything=w251) -> (data string=w250:string)  [unwired: 3 in, 2 out]
        n151 = call <vilib>:"Send Local Message.vi"("message queue in"=w255, "message name"="Write_Tag", "message value"=w250) -> ()  [unwired: 10 in, 3 out]
      }
      event "Suck Pump fraction of inflow": Value Change {
        n152 = event-data() -> ("NewVal"=w258:dbl)  [unwired: 1 out]
        n153 = Divide(x=w258, y=100.0) -> (x/y=w257:dbl)
        n154 = Number To Fractional String(number=w257) -> (F-format string=w260:string)  [unwired: 3 in]
        n155 = Bundle By Name(cluster=w266, "Data Type"=Data_Types."Double", "Name"="HMI_TNK5_SuckPmpFrac_Setpoint", "Value"=w260) -> (w263:T1)
        n156 = Flatten To String(anything=w263) -> (data string=w262:string)  [unwired: 3 in, 2 out]
        n157 = call <vilib>:"Send Local Message.vi"("message queue in"=w267, "message name"="Write_Tag", "message value"=w262) -> ()  [unwired: 10 in, 3 out]
      }
      event Menu Selection (User) {
        # "Add run-time menu items to the message\nqueue. The message handler case names must match the menu ItemTag names."
        n158 = event-data() -> ("ItemTag"=w270:string)  [unwired: 1 out]
        n159 = call <vilib>:"Send Local Message.vi"("message queue in"=w269, "message name"=w270) -> ()  [unwired: 11 in, 3 out]
      }
      event "Cell T Last Hr": Value Change {
        n160 = event-data() -> ("NewVal"=w272:bool)  [unwired: 3 out]
        n161 = case shown="True" w272 {
          tunnel: w271 -> [_ w275]
          frame False {
          }
          frame True {
            n162 = call <vilib>:"Send Local Message.vi"("message queue in"=w275, "message name"="DisplayLastHr", "message value"="TNK5_Temperature") -> ()  [unwired: 10 in, 3 out]
          }
        }
      }
      event "BasT1_Level Last Hr": Value Change {
        n163 = event-data() -> ("NewVal"=w277:bool)  [unwired: 3 out]
        n164 = case shown="True" w277 {
          tunnel: w276 -> [_ w280]
          frame False {
          }
          frame True {
            n165 = call <vilib>:"Send Local Message.vi"("message queue in"=w280, "message name"="DisplayLastHr", "message value"="BAS_Proc3_Tank_Level") -> ()  [unwired: 10 in, 3 out]
          }
        }
      }
      event "BasT1_P Last Hr": Value Change {
        n166 = event-data() -> ("NewVal"=w282:bool)  [unwired: 3 out]
        n167 = case shown="True" w282 {
          tunnel: w281 -> [_ w285]
          frame False {
          }
          frame True {
            n168 = call <vilib>:"Send Local Message.vi"("message queue in"=w285, "message name"="DisplayLastHr", "message value"="TNK56_MainPressure") -> ()  [unwired: 10 in, 3 out]
          }
        }
      }
      event "Supply Tot FlwLast Hr": Value Change {
        n169 = event-data() -> ("NewVal"=w287:bool)  [unwired: 3 out]
        n170 = case shown="True" w287 {
          tunnel: w286 -> [_ w290]
          frame False {
          }
          frame True {
            n171 = call <vilib>:"Send Local Message.vi"("message queue in"=w290, "message name"="DisplayLastHr", "message value"="Proc5_Total_Flow") -> ()  [unwired: 10 in, 3 out]
          }
        }
      }
      event "Suck FlwLast Hr": Value Change {
        n172 = event-data() -> ("NewVal"=w292:bool)  [unwired: 3 out]
        n173 = case shown="True" w292 {
          tunnel: w291 -> [_ w295]
          frame False {
          }
          frame True {
            n174 = call <vilib>:"Send Local Message.vi"("message queue in"=w295, "message name"="DisplayLastHr", "message value"="TNK5_SuckFlow") -> ()  [unwired: 10 in, 3 out]
          }
        }
      }
      event "Level Last Hr": Value Change {
        n175 = event-data() -> ("NewVal"=w297:bool)  [unwired: 3 out]
        n176 = case shown="True" w297 {
          tunnel: w296 -> [_ w300]
          frame False {
          }
          frame True {
            n177 = call <vilib>:"Send Local Message.vi"("message queue in"=w300, "message name"="DisplayLastHr", "message value"="TNK5_Level") -> ()  [unwired: 10 in, 3 out]
          }
        }
      }
      event "FlowControl Last Hr": Value Change {
        n178 = event-data() -> ("NewVal"=w302:bool)  [unwired: 3 out]
        n179 = case shown="True" w302 {
          tunnel: w301 -> [_ w305]
          frame False {
          }
          frame True {
            n180 = call <vilib>:"Send Local Message.vi"("message queue in"=w305, "message name"="DisplayLastHr", "message value"="TNK5_ProcVlv1_ActlPos") -> ()  [unwired: 10 in, 3 out]
          }
        }
      }
      event "Flow 1 Last Hr": Value Change {
        n181 = event-data() -> ("NewVal"=w307:bool)  [unwired: 3 out]
        n182 = case shown="True" w307 {
          tunnel: w306 -> [_ w310]
          frame False {
          }
          frame True {
            n183 = call <vilib>:"Send Local Message.vi"("message queue in"=w310, "message name"="DisplayLastHr", "message value"="TNK5_Flow1") -> ()  [unwired: 10 in, 3 out]
          }
        }
      }
      event "Flow 2 Last Hr": Value Change {
        n184 = event-data() -> ("NewVal"=w312:bool)  [unwired: 3 out]
        n185 = case shown="True" w312 {
          tunnel: w311 -> [_ w315]
          frame False {
          }
          frame True {
            n186 = call <vilib>:"Send Local Message.vi"("message queue in"=w315, "message name"="DisplayLastHr", "message value"="TNK5_Flow2") -> ()  [unwired: 10 in, 3 out]
          }
        }
      }
      event "Flow 3 Last Hr": Value Change {
        n187 = event-data() -> ("NewVal"=w317:bool)  [unwired: 3 out]
        n188 = case shown="True" w317 {
          tunnel: w316 -> [_ w320]
          frame False {
          }
          frame True {
            n189 = call <vilib>:"Send Local Message.vi"("message queue in"=w320, "message name"="DisplayLastHr", "message value"="TNK5_Flow3") -> ()  [unwired: 10 in, 3 out]
          }
        }
      }
      event "Flow 4 Last Hr": Value Change {
        n190 = event-data() -> ("NewVal"=w322:bool)  [unwired: 3 out]
        n191 = case shown="True" w322 {
          tunnel: w321 -> [_ w325]
          frame False {
          }
          frame True {
            n192 = call <vilib>:"Send Local Message.vi"("message queue in"=w325, "message name"="DisplayLastHr", "message value"="TNK5_Flow4") -> ()  [unwired: 10 in, 3 out]
          }
        }
      }
      event "Rectifer Settings": Mouse Down {
        n193 = event-data() -> ("CtlRef"=w332:refnum<vi>, "Coords"=w330:T7, "Button"=w331:u16)  [unwired: 6 out]
        n194 = call "Handle Rectifer Step Selection.vi"("Coords"=w330, "Button"=w331, "MulticolumnListbox in"=w332) -> ("Row"=w326:i32)  [unwired: 8 in]
        n195 = Greater Than 0?(x=w326) -> (x > 0?=w329:bool)
        n196 = case shown="True" w329 {
          tunnel: w328 -> [_ w335]
          tunnel: w327 -> [_ w334]
          tunnel: w326 -> [_ w333]
          frame False {
          }
          frame True {
            n197 = Number To Decimal String(number=w333) -> (decimal integer string=w336:string)  [unwired: 1 in]
            n198 = Bundle By Name(cluster=w334, "Data Type"=Data_Types."I32", "Name"="HMI_Rect9_10_NumSteps", "Value"=w336) -> (w340:T1)
            n199 = Flatten To String(anything=w340) -> (data string=w339:string)  [unwired: 3 in, 2 out]
            n200 = call <vilib>:"Send Local Message.vi"("message queue in"=w335, "message name"="Write_Tag", "message value"=w339) -> ("message queue out"=w338:T5)  [unwired: 10 in, 2 out]
            n201 = call <vilib>:"Send Local Message.vi"("message queue in"=w338, "message name"="UpdatePlatingMinutes", "message value"=w336) -> ()  [unwired: 10 in, 3 out]
          }
        }
      }
      event "Rectifer Settings": Edit Cell {
        n202 = event-data() -> ("CtlRef"=w350:refnum<vi>, "String"=w349:string, "Coords"=w348:T8)  [unwired: 4 out]
        n203 = call "Data Check Rectifier Settings.vi"("String"=w349, "Coords"=w348, "MulticolumnListbox in"=w350) -> ("error out"=w345:errorcluster)  [unwired: 7 in, 1 out]
        n204 = shared-variable-read(refnum<k21> "ni.var.psp://z004551/CDL0100 ReadWriteTags/HMI_Rect9_10_NumSteps" ("shared variable refnum in"), 0) -> (w351:i32)  [unwired: 1 in, 3 out]
        n205 = Number To Decimal String(number=w351) -> (decimal integer string=w344:string)  [unwired: 1 in]
        n206 = call <vilib>:"Send Local Message.vi"("message queue in"=w346, "message name"="UpdatePlatingMinutes", "message value"=w344, "error in"=w345) -> ()  [unwired: 9 in, 3 out]
      }
      event "MO": Value Change {
        n207 = event-data() -> ("NewVal"=w354:string)  [unwired: 6 out]
        n208 = shared-variable ".\\Local Variables.lvlib\\PT5_MO"(w354) -> ()  [unwired: 1 in, 1 out]
      }
    }
  }
  n209 = while "Message Processor" {
    shift-left: w2 -> [w364]
    shift-right: [w368] -> w8
    tunnel: w20 -> [w365]
    tunnel: w15 -> [w359]
    tunnel: [w359] -> w9
    shift-right: [w356] -> _
    shift-left: w7 -> [w357]
    tunnel: w1 -> [w355]
    stop <- w367 stop-if-true
    w360 = 100  # Timeout
    n210 = call <vilib>:"Read Next Message.vi"("message queue in"=w365, "timeout (1 ms)"=w360, "error in"=w364) -> ("exit process?"=w367:bool, "message queue out"=w366:T5, "message name"=w362:string, "message value"=w361:string, "error out"=w363:errorcluster)  [unwired: 5 in, 3 out]
    n211 = case shown="\"Load_A_Recipe\"" w362 {
      selector: w362 -> [_ _ w460 _ _ _ _ _ _ _ _ _ _ _]
      tunnel: w366 -> [_ _ _ _ _ _ w612 _ _ _ _ w634 _ w658]
      tunnel: w363 -> [w369 w381 w461 w462 w464 w466 w613 w615 w619 w622 w624 w638 w652 w669]
      tunnel: [w369 w381 w461 errorcluster {"status"=FALSE, "code"=0, "source"=""} ("error out") w464 w466 w611 w615 w618 w622 w624 w637 w643 w661] -> w368
      tunnel: w361 -> [_ _ _ _ _ _ _ _ w617 _ w626 w629 _ _]
      tunnel: w359 -> [_ _ _ _ _ _ _ _ w620 _ _ _ _ _]
      tunnel: T1 {"Data Type"=enum."Double", "Name"="test", "Value"="", "Description"=""} ("Tag") -> [_ _ _ _ _ _ _ _ _ _ _ _ _ _]
      tunnel: w357 -> [_ w376 _ _ _ w465 _ _ w616 w623 w625 _ w642 w660]
      tunnel: [_ w377 _ _ _ w465 _ _ w616 w623 w625 _ w642 w660] -> w356
      tunnel: w355 -> [_ _ _ _ _ _ _ _ _ _ _ _ _ w659]
      frame "---------- Framework Operations ----------" {
        # "Dummy case to add a seperator in the Case Structure menu"
      }
      frame "", "Idle" {
        n212 = stacked-sequence {
          frame #0 {
            n213 = control-ref of="Enable Plating Cell"() -> (w387:refnum<vi>)
            n214 = shared-variable-read(refnum<k21> "ni.var.psp://z004551/CDL0100 ReadTags/Tnk5_Can_Plate" ("shared variable refnum in"), FALSE) -> (w397:bool)  [unwired: 1 in, 3 out]
            n215 = shared-variable-read(refnum<k21> "ni.var.psp://z004551/CDL0100 ReadWriteTags/HMI_Tank5_Enable" ("shared variable refnum in"), FALSE) -> (w384:bool)  [unwired: 1 in, 3 out]
            n216 = shared-variable-read(refnum<k21> "ni.var.psp://z004551/CDL0100 ReadWriteTags/HMI_Enable_BTnk3_Pump" ("shared variable refnum in"), FALSE) -> (w389:bool)  [unwired: 1 in, 3 out]
            n217 = shared-variable-read(refnum<k21> "ni.var.psp://z004551/CDL0100 ReadWriteTags/HMI_Tank6_Enable" ("shared variable refnum in"), FALSE) -> (w383:bool)  [unwired: 1 in, 3 out]
            n218 = Or(x=w384, y=w383) -> (x .or. y?=w382:bool)
            n219 = Or(x=w382, y=w389) -> (x .or. y?=w392:bool)
            n220 = case shown="False" w397 {
              tunnel: [T9."Disabled and Grayed Out" ("Disabled") T9."Enabled" ("Disabled")] -> w398
              frame False {
              }
              frame True {
              }
            }
            n221 = call "GrayOutButtonFromPSPVar.vi"("shared variable refnum in"=refnum<k21> "ni.var.psp://z004551/CDL0100 ReadWriteTags/HMI_Tank5_Drain", "Boolean in"=w387) -> ()  [unwired: 10 in]
            n222 = case shown="True" w392 {
              tunnel: [T9."Enabled" ("Disabled") T9."Disabled and Grayed Out" ("Disabled")] -> w391
              frame False {
              }
              frame True {
              }
            }
            n223 = control-ref of="Full Drain Plating Cell"() -> (w390:refnum<vi>)
            n224 = control-ref of="Start Cycle"() -> (w399:refnum<vi>)
            n225 = property class="Bool (strict)"(reference=w399, "DisabledEnum"=w398) -> ()  [unwired: 1 in, 2 out]
            n226 = property class="Bool (strict)"(reference=w390, "DisabledEnum"=w391) -> ()  [unwired: 1 in, 2 out]
          }
          frame #1 {
            n227 = shared-variable-read(refnum<k21> "ni.var.psp://z004551/CDL0100 ReadTags/IO_Bas_Tnk3_3Way_At_Recirc" ("shared variable refnum in"), FALSE) -> (w409:bool)  [unwired: 1 in, 3 out]
            n228 = shared-variable-read(refnum<k21> "ni.var.psp://z004551/CDL0100 ReadTags/IO_Bas_Tnk3_3Way_At_Open" ("shared variable refnum in"), FALSE) -> (w410:bool)  [unwired: 1 in, 3 out]
            n229 = shared-variable-read(refnum<k21> "ni.var.psp://z004551/CDL0100 ReadTags/IO_Bas_Tnk3_3Way_At_Closed" ("shared variable refnum in"), FALSE) -> (w413:bool)  [unwired: 1 in, 3 out]
            n230 = Or(x=w410, y=w409) -> (x .or. y?=w407:bool)
            "Sump Return" <- w407
            "Boolean 2" <- w407
            n231 = Or(x=w413, y=w410) -> (x .or. y?=w408:bool)
            "Return to sump" <- w408
            "Drain Tee Top" <- w408
            "Return to sump 2" <- w408
            "Process 1 Supply" <- w408
            n232 = Or(x=w408, y=w407) -> (x .or. y?=→"Boolean 5":bool)
          }
          frame #2 {
            n233 = shared-variable-read(refnum<k21> "ni.var.psp://z004551/CDL0100 ReadWriteTags/HMI_Tank5_Drain" ("shared variable refnum in"), FALSE) -> (w418:bool)  [unwired: 1 in, 3 out]
            n234 = shared-variable-read(refnum<k21> "ni.var.psp://z004551/CDL0100 ReadWriteTags/HMI_Enable_BTnk3_Pump" ("shared variable refnum in"), FALSE) -> (w419:bool)  [unwired: 1 in, 3 out]
            n235 = Or(x=w419, y=w418) -> (x .or. y?=→"SumpBottom":bool)
          }
          frame #3 {
            n236 = shared-variable-read(refnum<k21> "ni.var.psp://z004551/CDL0100 ReadTags/Rect9_10_CurrRecpStp" ("shared variable refnum in"), 0) -> (w425:i32)  [unwired: 1 in, 3 out]
            n237 = call-poly <userlib>:"Data Changed__ogtk.vi"("I32"=w425) -> ("Changed"=w426:bool)
            n238 = case shown="True" w426 {
              tunnel: w425 -> [_ w430]
              frame False {
              }
              frame True {
                w435 = 0.0 ("Scale.Range:Minimum")
                n239 = shared-variable-read(refnum<k21> "ni.var.psp://z004551/CDL0100 ReadWriteTags/HMI_Rect9_10_NumSteps" ("shared variable refnum in"), 0) -> (w429:i32)  [unwired: 1 in, 3 out]
                n240 = Less?(x=w430, y=w429) -> (x < y?=w442:bool)
                n241 = case shown="False" w442 {
                  tunnel: w430 -> [w447 w448]
                  tunnel: [w446 w448] -> w436
                  frame False {
                    n242 = Decrement(x=w447) -> (x-1=w446:i32)
                  }
                  frame True {
                  }
                }
                n243 = shared-variable-read(refnum<k21> "ni.var.psp://z004551/CDL0100 ReadWriteTags/HMI_Rct10_AMin_SetPnts" ("shared variable refnum in"), dbl[] []) -> (w437:dbl[])  [unwired: 1 in, 3 out]
                n244 = Index Array(array=w437, index=w436) -> (element=w433:dbl)
                n245 = shared-variable-read(refnum<k21> "ni.var.psp://z004551/CDL0100 ReadWriteTags/HMI_Rct9_AMin_SetPnts" ("shared variable refnum in"), dbl[] []) -> (w440:dbl[])  [unwired: 1 in, 3 out]
                n246 = Index Array(array=w440, index=w436) -> (element=w434:dbl)
                n247 = control-ref of="Right Anode Amp-min"() -> (w432:refnum<vi>)
                n248 = control-ref of="Left Anode Amp-min"() -> (w431:refnum<vi>)
                n249 = property class="Slide (strict)"(reference=w431, "Scale.Maximum"=w434, "Scale.Minimum"=w435) -> ()  [unwired: 1 in, 2 out]
                n250 = property class="Slide (strict)"(reference=w432, "Scale.Maximum"=w433, "Scale.Minimum"=w435) -> ()  [unwired: 1 in, 2 out]
              }
            }
          }
        }
        n251 = local read "Left Output On"() -> (w373:bool)
        n252 = local read "Right Output On"() -> (w374:bool)
        n253 = control-ref of="status"() -> (w380:refnum<vi>)
        n254 = Tick Count (ms)() -> (millisecond timer value=w375:u32)
        n255 = Subtract(x=w375, y=w376) -> (x-y=w378:u32)
        n256 = call <userlib>:"TAE Format Alarm Ticker.vi"("Alarm Ticker Ref"=w380) -> ()  [unwired: 15 in]
        n257 = Or(x=w373, y=w374) -> (x .or. y?=w372:bool)
        n258 = Greater?(x=w378, y=u32 500) -> (0:w371:bool)
        n259 = And(x=w372, y=w371) -> (x .and. y?=w370:bool)
        n260 = case shown="True" w370 {
          tunnel: w375 -> [_ w450]
          tunnel: [w449 w450] -> w377
          tunnel: w376 -> [w449 _]
          frame False {
          }
          frame True {
            n261 = shared-variable-read(refnum<k21> "ni.var.psp://z004551/CDL0100 ReadTags/Rect9_ActlVolts" ("shared variable refnum in"), 0.0) -> (w453:dbl)  [unwired: 1 in, 3 out]
            n262 = shared-variable-read(refnum<k21> "ni.var.psp://z004551/CDL0100 ReadTags/Rect10_ActlVolts" ("shared variable refnum in"), 0.0) -> (w452:dbl)  [unwired: 1 in, 3 out]
            n263 = Bundle(w453, w452) -> (→"Output Voltage":cluster{dbl, dbl})  [unwired: 1 in]
          }
        }
      }
      frame "Missing Message Handler", Default {
        # "Call this case if a message is received that is not handled \nby any other case. Typically this is a programming error\nas a result of a typo or unhandled message/missing message handler."
        n264 = Format Into String(format string="DevError: Missing message handler for '%s\" message." ("message"), w460) -> (resulting string=w458:string)  [unwired: 2 in, 1 out]
        n265 = One Button Dialog(message=w458) -> ()  [unwired: 2 out]
      }
      frame "Error" {
        # "General Error Case - this case is called if an error is passed using the error cluster below. Typically most new errors should be handed in each individual case and not passed in the rror cluster. If necessary a custom error handler case should be added and called from other cases."
        n266 = call <vilib>:"Simple Error Handler.vi"("error in (no error)"=w462) -> ()  [unwired: 1 in, 8 out]
      }
      frame "---------- Generic Operations ----------" {
        # "Dummy case to add a seperator in the Case Structure menu"
      }
      frame "Initialize" {
        n267 = stacked-sequence {
          seq-local: [_ w487 _ _ _ _] -> [_ _ w506 _ w550 w590]
          seq-local: [_ _ w504 _ _ _] -> [_ _ _ _ w545 w598]
          seq-local: [_ _ w503 _ _ _] -> [_ _ _ _ w543 w593]
          seq-local: [_ _ _ w534 _ _] -> [_ _ _ _ w544 _]
          seq-local: [_ _ _ w525 _ _] -> [_ _ _ _ w542 _]
          seq-local: [_ _ _ w524 _ _] -> [_ _ _ _ w541 _]
          seq-local: [_ _ _ w523 _ _] -> [_ _ _ _ w540 _]
          seq-local: [_ _ _ w522 _ _] -> [_ _ _ _ w539 _]
          frame #0 {
            n268 = shared-variable-read(refnum<k21> "ni.var.psp://z004551/CDL0100 ReadWriteTags/HMI_TNK5_SuckPmpFrac_Setpoint" ("shared variable refnum in"), 0.0) -> (w472:dbl)  [unwired: 1 in, 3 out]
            n269 = shared-variable-read(refnum<k21> "ni.var.psp://z004551/CDL0100 ReadWriteTags/HMI_Tnk5_Enable_SuckPump" ("shared variable refnum in"), FALSE) -> (w475:bool)  [unwired: 1 in, 3 out]
            n270 = shared-variable-read(refnum<k21> "ni.var.psp://z004551/CDL0100 ReadWriteTags/HMI_Tnk5_Rack_RPM" ("shared variable refnum in"), 0.0) -> (w486:dbl)  [unwired: 1 in, 3 out]
            n271 = shared-variable-read(refnum<k21> "ni.var.psp://z004551/CDL0100 ReadWriteTags/HMI_Tank5_Rack_Motor_Run" ("shared variable refnum in"), FALSE) -> (w485:bool)  [unwired: 1 in, 3 out]
            n272 = shared-variable-read(refnum<k21> "ni.var.psp://z004551/CDL0100 ReadWriteTags/HMI_Tank5_Motion_OverRide" ("shared variable refnum in"), FALSE) -> (w467:bool)  [unwired: 1 in, 3 out]
            n273 = shared-variable-read(refnum<k21> "ni.var.psp://z004551/CDL0100 ReadWriteTags/HMI_TNK5_Flow_Setpoint" ("shared variable refnum in"), 0.0) -> (w484:dbl)  [unwired: 1 in, 3 out]
            n274 = Multiply(x=w472, y=100.0) -> (x*y=w470:dbl)
            n275 = local write "Enable Suck Pump"(w475) -> ()
            n276 = local write "Rack RPM"(w486) -> ()
            n277 = local write "Enable Rack Motion"(w485) -> ()
            n278 = local write "Total Inflow (L/min)"(w484) -> ()
            n279 = local write "Suck Pump fraction of inflow"(w470) -> ()
            n280 = local write "Override Motion"(w467) -> ()
          }
          frame #1 {
            n281 = shared-variable-read(refnum<k21> "ni.var.psp://z004551/CDL0100 ReadWriteTags/HMI_Tank5_Drain" ("shared variable refnum in"), FALSE) -> (w490:bool)  [unwired: 1 in, 3 out]
            n282 = shared-variable-read(refnum<k21> "ni.var.psp://z004551/CDL0100 ReadWriteTags/HMI_Tnk5_Eductor_RPM" ("shared variable refnum in"), 0.0) -> (w498:dbl)  [unwired: 1 in, 3 out]
            n283 = shared-variable-read(refnum<k21> "ni.var.psp://z004551/CDL0100 ReadWriteTags/HMI_Tank5_Enable" ("shared variable refnum in"), FALSE) -> (w497:bool)  [unwired: 1 in, 3 out]
            n284 = local write "Full Drain Plating Cell"(w490) -> ()
            n285 = shared-variable-read(refnum<k21> "ni.var.psp://z004551/CDL0100 ReadWriteTags/HMI_Tank5_Eductor_Motors_Run" ("shared variable refnum in"), FALSE) -> (w501:bool)  [unwired: 1 in, 3 out]
            n286 = shared-variable-read(refnum<k21> "ni.var.psp://z004551/CDL0100 ReadWriteTags/HMI_Rect9_10_NumSteps" ("shared variable refnum in"), 0) -> (w487:i32)  [unwired: 1 in, 3 out]
            n287 = local write "Enable Plating Cell"(w497) -> ()
            n288 = local write "Eductor RPM"(w498) -> ()
            n289 = local write "Enable Eductor Motion"(w501) -> ()
          }
          frame #2 {
            w507 = 0.0
            n290 = shared-variable ".\\Local Variables.lvlib\\PT5_MO"() -> (w502:string)  [unwired: 1 in, 1 out]
            n291 = shared-variable-read(refnum<k21> "ni.var.psp://z004551/CDL0100 ReadWriteTags/HMI_Rct9_AMin_SetPnts" ("shared variable refnum in"), dbl[] []) -> (w504:dbl[])  [unwired: 1 in, 3 out]
            n292 = shared-variable-read(refnum<k21> "ni.var.psp://z004551/CDL0100 ReadWriteTags/HMI_Rct10_AMin_SetPnts" ("shared variable refnum in"), dbl[] []) -> (w503:dbl[])  [unwired: 1 in, 3 out]
            n293 = shared-variable-read(refnum<k21> "ni.var.psp://z004551/CDL0100 ReadWriteTags/HMI_BAS_TNK3_P_Setpoint" ("shared variable refnum in"), 0.0) -> (w513:dbl)  [unwired: 1 in, 3 out]
            n294 = for {
              N: w506 -> [_]
              tunnel: w503 -> [w518] mode=indexing
              shift-right: [w516] -> w505
              shift-left: w507 -> [w517]
              n295 = Add(x=w518, y=w517) -> (x+y=w516:dbl)
            }
            n296 = for {
              N: w506 -> [_]
              tunnel: w504 -> [w521] mode=indexing
              shift-right: [w519] -> w510
              shift-left: w507 -> [w520]
              n297 = Add(x=w521, y=w520) -> (x+y=w519:dbl)
            }
            n298 = local write "Supply Pressure (kPa)"(w513) -> ()
            n299 = local write "MO"(w502) -> ()
            n300 = local write "Total Amp*min L"(w510) -> ()
            n301 = local write "Total Amp*min R"(w505) -> ()
          }
          frame #3 {
            n302 = shared-variable-read(refnum<k21> "ni.var.psp://z004551/CDL0100 ReadWriteTags/HMI_Rct10_AFwd_SetPnts" ("shared variable refnum in"), dbl[] []) -> (w534:dbl[])  [unwired: 1 in, 3 out]
            n303 = shared-variable-read(refnum<k21> "ni.var.psp://z004551/CDL0100 ReadWriteTags/HMI_Rct9_FwdOffTm_SetPnts" ("shared variable refnum in"), dbl[] []) -> (w524:dbl[])  [unwired: 1 in, 3 out]
            n304 = shared-variable-read(refnum<k21> "ni.var.psp://z004551/CDL0100 ReadWriteTags/HMI_Rct9_FwdTm_SetPnts" ("shared variable refnum in"), dbl[] []) -> (w525:dbl[])  [unwired: 1 in, 3 out]
            n305 = shared-variable-read(refnum<k21> "ni.var.psp://z004551/CDL0100 ReadWriteTags/HMI_Rct9_BwdTm_SetPnts" ("shared variable refnum in"), dbl[] []) -> (w523:dbl[])  [unwired: 1 in, 3 out]
            n306 = shared-variable-read(refnum<k21> "ni.var.psp://z004551/CDL0100 ReadWriteTags/HMI_Rct9_BwdOffTm_SetPnts" ("shared variable refnum in"), dbl[] []) -> (w522:dbl[])  [unwired: 1 in, 3 out]
          }
          frame #4 {
            n307 = Subtract(x=10, y=w550) -> (x-y=w553:i32)
            n308 = Initialize Array(38, w550) -> (w552:i32[])
            n309 = Initialize Array(37, w553) -> (w551:i32[])
            n310 = Build Array (concatenate)(w552, w551) -> (w548:i32[])
            n311 = shared-variable-read(refnum<k21> "ni.var.psp://z004551/CDL0100 ReadWriteTags/HMI_Rct9_AFwd_SetPnts" ("shared variable refnum in"), dbl[] []) -> (w547:dbl[])  [unwired: 1 in, 3 out]
            n312 = for {
              N: 10 -> [_]
              tunnel: [w588] -> w538 mode=indexing
              tunnel: [w586] -> w537 mode=indexing
              tunnel: w547 -> [w584] mode=indexing
              tunnel: w545 -> [w581] mode=indexing
              tunnel: w544 -> [w578] mode=indexing
              tunnel: w543 -> [w575] mode=indexing
              tunnel: w542 -> [w572] mode=indexing
              tunnel: w541 -> [w569] mode=indexing
              tunnel: w540 -> [w566] mode=indexing
              tunnel: w539 -> [w563] mode=indexing
              i -> [w560]
              n313 = Number To Fractional String(number=w572, precision (6)=i16 1) -> (F-format string=w571:string)  [unwired: 2 in]
              n314 = Number To Fractional String(number=w575, precision (6)=i16 1) -> (F-format string=w574:string)  [unwired: 2 in]
              n315 = Number To Fractional String(number=w581, precision (6)=i16 1) -> (F-format string=w580:string)  [unwired: 2 in]
              n316 = Number To Fractional String(number=w578, precision (6)=i16 1) -> (F-format string=w577:string)  [unwired: 2 in]
              n317 = Number To Fractional String(number=w584, precision (6)=i16 1) -> (F-format string=w583:string)  [unwired: 2 in]
              n318 = Number To Fractional String(number=w569, precision (6)=i16 1) -> (F-format string=w568:string)  [unwired: 2 in]
              n319 = Number To Fractional String(number=w566, precision (6)=i16 1) -> (F-format string=w565:string)  [unwired: 2 in]
              n320 = Increment(x=w560) -> (x+1=w559:i32)
              n321 = Number To Decimal String(number=w560) -> (decimal integer string=w588:string)  [unwired: 1 in]
              n322 = Number To Fractional String(number=w563, precision (6)=i16 1) -> (F-format string=w562:string)  [unwired: 2 in]
              n323 = call "Build Text"("d"=w559) -> ("Result"=w561:string)  [unwired: 13 in, 1 out]
              n324 = Build Array("Active", w583, w580, w577, w574, w571, w568, w565, w562, w561) -> (w586:string[])
            }
            n325 = control-ref of="Rectifer Settings"() -> (w549:refnum<vi>)
            n326 = property class="MCListbox (strict)"(reference=w549, "ItemSyms"=w548, "RowHdrs[]"=w538, "ItemNames"=w537) -> ()  [unwired: 1 in, 2 out]
          }
          frame #5 {
            n327 = control-ref of="Rectifer Settings"() -> (w607:refnum<vi>)
            n328 = control-ref of="Right Anode Amp-min"() -> (w599:refnum<vi>)
            n329 = control-ref of="Left Anode Amp-min"() -> (w600:refnum<vi>)
            n330 = local read "Reverse Current Multiplier"() -> (w589:dbl)
            n331 = property class="MCListbox (strict)"(reference=w607) -> ("ItemNames"=w606:string[][])  [unwired: 1 in, 2 out]
            n332 = shared-variable-read(refnum<k21> "ni.var.psp://z004551/CDL0100 ReadTags/Rect9_10_CurrRecpStp" ("shared variable refnum in"), 0) -> (w591:i32)  [unwired: 1 in, 3 out]
            n333 = call "Calculate Plating Time.vi"("Num Steps"=w590, "ItemNames"=w606, "Reverse Current Multiplier"=w589) -> ("Right Anode Time"=w604:dbl, "Left Anode Time"=w605:dbl)  [unwired: 7 in]
            n334 = Less?(x=w591, y=w590) -> (x < y?=w601:bool)
            n335 = case shown="False" w601 {
              tunnel: w591 -> [w609 w610]
              tunnel: [w608 w610] -> w594
              frame False {
                n336 = Decrement(x=w609) -> (x-1=w608:i32)
              }
              frame True {
              }
            }
            n337 = local write "Right Time"(w604) -> ()
            n338 = local write "Left Time"(w605) -> ()
            n339 = Index Array(array=w598, index=w594) -> (element=w597:dbl)
            n340 = Index Array(array=w593, index=w594) -> (element=w592:dbl)
            n341 = property class="Slide (strict)"(reference=w600, "Scale.Maximum"=w597, "Scale.Minimum"=0.0 ("Scale.Range:Minimum")) -> ()  [unwired: 1 in, 2 out]
            n342 = property class="Slide (strict)"(reference=w599, "Scale.Maximum"=w592, "Scale.Minimum"=0.0 ("Scale.Range:Minimum")) -> ()  [unwired: 1 in, 2 out]
          }
        }
      }
      frame "Exit" {
        # "Destroy message queue >> this will halt the UI event handler loop"
        # "Stop the VI\n>> Perform any cleanup tasks in this message case.\n>> Clear display before closing."
        n343 = call <vilib>:"Destroy Message Queue.vi"("message queue in"=w612, "error in"=w613) -> ("error out"=w611:errorcluster)  [unwired: 11 in, 2 out]
        n344 = local write "status"("" ("Status")) -> ()
      }
      frame "---------- Application Operations ----------" {
        # "Dummy case to add a seperator in the Case Structure menu"
      }
      frame "Write_Tag" {
        n345 = call-poly <vilib>:"Write Message.vi"("error in"=w619, "data"=w617, "name"="WriteTag", "connection info in"=w620) -> ("error out"=w618:errorcluster)  [unwired: 6 in, 1 out]
      }
      frame "UpdateVPlotX" {
      }
      frame "DisplayLastHr" {
        n346 = call "Trace Variable 1 hour Popup.vi"("Tag"=w626) -> ()  [unwired: 11 in]
      }
      frame "UpdatePlatingMinutes" {
        n347 = local read "Reverse Current Multiplier"() -> (w627:dbl)
        n348 = Decimal String To Number(string=w629) -> (number=w628:i32)  [unwired: 2 in, 1 out]
        n349 = control-ref of="Rectifer Settings"() -> (w635:refnum<vi>)
        n350 = call "Assemble Rectifier Setting Changes for PLC.vi"("Num Steps"=w628, "Rect Number"=9, "error In"=w638, "Reverse Current Multiplier"=w627, "message queue in"=w634, "MulticolumnListbox in"=w635) -> ("Right Anode Mins"=w630:dbl, "Left Anode Mins"=w631:dbl, "Right AmpMin"=w632:dbl, "Left AmpMin"=w633:dbl, "error out"=w637:errorcluster)  [unwired: 1 in]
        n351 = local write "Total Amp*min L"(w633) -> ()
        n352 = local write "Total Amp*min R"(w632) -> ()
        n353 = local write "Left Time"(w631) -> ()
        n354 = local write "Right Time"(w630) -> ()
      }
      frame "Save_Recipe" {
        n355 = control-ref of="Rectifer Settings"() -> (w653:refnum<vi>)
        n356 = local read "Reverse Current Multiplier"() -> (w641:dbl)
        n357 = call "Convert RectifierListData to Arrays.vi"("MulticolumnListbox in"=w653, "error in (no error)"=w652) -> ("Left Amps"=w649:dbl[], "Right Amps"=w648:dbl[], "Left AmpMins"=w646:dbl[], "Right Amp Min"=w645:dbl[], "error out"=w644:errorcluster)  [unwired: 5 in, 4 out]
        n358 = shared-variable-read(refnum<k21> "ni.var.psp://z004551/CDL0100 ReadWriteTags/HMI_Rect9_10_NumSteps" ("shared variable refnum in"), 0) -> (w647:i32)  [unwired: 1 in, 3 out]
        n359 = call "Save Rectifier Recipe.vi"("Rev Mult"=w641, "Right AmpMins"=w645, "Left AmpMins"=w646, "error in"=w644, "Number Steps"=w647, "Right Amps"=w648, "Left Amps"=w649) -> ("error out"=w643:errorcluster, "name"=w639:string, "cancelled"=w640:bool)  [unwired: 2 in]
        n360 = case shown="False" w640 {
          tunnel: w639 -> [w654 _]
          frame False {
            n361 = local write "Loaded Recipe"(w654) -> ()
          }
          frame True {
          }
        }
      }
      frame "Load_A_Recipe" {
        n362 = call "BrowseRecipe.vi"() -> ("selected path"=w655:path)  [unwired: 9 in, 2 out]
        n363 = call "Read Rectifier Recipe.vi"("selected path"=w655, "error in"=w669) -> ("Left Amps"=w666:dbl[], "Left AmpMins"=w665:dbl[], "Canceled?"=w668:bool, "Num Steps"=w667:i32, "name"=w656:string, "Rev Mult"=w657:dbl, "Right Amps"=w664:dbl[], "Right AmpMins"=w662:dbl[], "error out"=w663:errorcluster)  [unwired: 5 in]
        n364 = case shown="False" w668 {
          tunnel: w667 -> [w676 _]
          tunnel: w666 -> [w690 _]
          tunnel: w665 -> [w689 _]
          tunnel: w664 -> [w688 _]
          tunnel: w663 -> [w687 w692]
          tunnel: w662 -> [w686 _]
          tunnel: [w672 w692] -> w661
          tunnel: w659 -> [w677 _]
          tunnel: w658 -> [w675 _]
          tunnel: w657 -> [w671 _]
          tunnel: w656 -> [w670 _]
          frame False {
            n365 = local write "Loaded Recipe"(w670) -> ()
            n366 = control-ref of="Rectifer Settings"() -> (w691:refnum<vi>)
            n367 = call "Write Pulse Rectifier Recipe to ListBox.vi"("Right AmpMins"=w686, "Left AmpMins"=w689, "Right Amps"=w688, "Left Amps"=w690, "error in (no error)"=w687, "Number Steps"=w676, "ListBox"=w691) -> ("error out"=w674:errorcluster)  [unwired: 4 in]
            n368 = local write "Reverse Current Multiplier"(w671) -> ()
            n369 = Number To Decimal String(number=w676) -> (decimal integer string=w678:string)  [unwired: 1 in]
            n370 = Bundle By Name(cluster=w677, "Data Type"=Data_Types."I32", "Name"="HMI_Rect9_10_NumSteps", "Value"=w678) -> (w682:T1)
            n371 = Flatten To String(anything=w682) -> (data string=w681:string)  [unwired: 3 in, 2 out]
            n372 = call <vilib>:"Send Local Message.vi"("message queue in"=w675, "message name"="Write_Tag", "message value"=w681, "error in"=w674) -> ("message queue out"=w680:T5, "error out"=w673:errorcluster)  [unwired: 9 in, 1 out]
            n373 = call <vilib>:"Send Local Message.vi"("message queue in"=w680, "message name"="UpdatePlatingMinutes", "message value"=w678, "error in"=w673) -> ("error out"=w672:errorcluster)  [unwired: 9 in, 2 out]
          }
          frame True {
          }
        }
      }
    }
  }
  n374 = call-poly <vilib>:"Get Connection Reference.vi"("error in"=w8, "connection info in"=w9) -> ("error out"=w12:errorcluster, "connection ID out"=w11:refnum<k5>)  [unwired: 8 out]
  n375 = TCP Close Connection(connection ID=w11, error in (no error)=w12) -> (error out=w14:errorcluster)  [unwired: 2 out]
  n376 = call <vilib>:"Error to Warning.vi"("1st Error to Convert"=w13, "error in"=w14) -> ("warning out"=w10:errorcluster)  [unwired: 3 in, 10 out]
  n377 = call <vilib>:"Simple Error Handler.vi"("error in (no error)"=w10) -> ()  [unwired: 4 in, 5 out]
